vi "SS2 Live_Get PCB Version.vi"(8 "error in (no error)":errorcluster, 11 "serialNumber":string) -> (0 "error out":errorcluster, 2 "PCB Version":T1, 3 "serialNumber (dup)":string)   [LabVIEW 2019]
uses:
  SS2 DAQ PCB Version.ctl
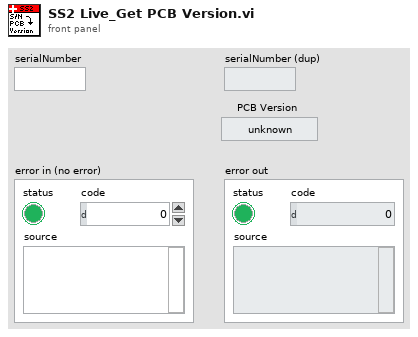
[diagram p1: front panel]
types:
  T1 = typedef "SS2 DAQ PCB Version.ctl" = enum16{"unknown", "PCB 1", "PCB 2"}
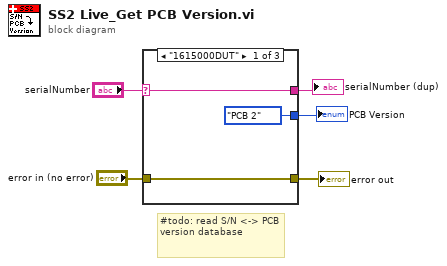
[diagram p0: block diagram]
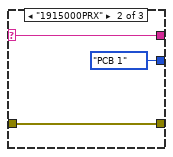
[diagram p2: hidden frame]
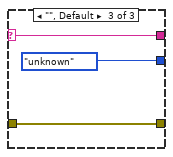
[diagram p3: hidden frame]
diagram:
  # "#todo: read S/N <-> PCB version database"
  n1 = case shown="\"1615000DUT\"" "serialNumber" {
    selector: "serialNumber" -> [w6 w9 w14]
    tunnel: [w8 w11 w12] -> w4
    tunnel: [w6 w9 w14] -> w2
    tunnel: [SS2_DAQ_PCB_Version."PCB 2" ("PCB Version") SS2_DAQ_PCB_Version."PCB 1" ("PCB Version") SS2_DAQ_PCB_Version."unknown" ("PCB Version")] -> w1
    tunnel: "error in (no error)" -> [w8 w11 w12]
    frame "1615000DUT" {
    }
    frame "1915000PRX" {
    }
    frame "", Default {
    }
  }
  "PCB Version" <- w1
  "serialNumber (dup)" <- w2
  "error out" <- w4
